vi "Serial_Port_Select.vi"(8 "error in":errorcluster, 11 "PortString":string) -> (0 "error out":errorcluster, 2 "SelectedPort":string, 3 "PortList":string[](array[string]))   [LabVIEW 2020]
uses:
  <vilib>/Instr/_visa.llb/VISA Find Search Mode.ctl
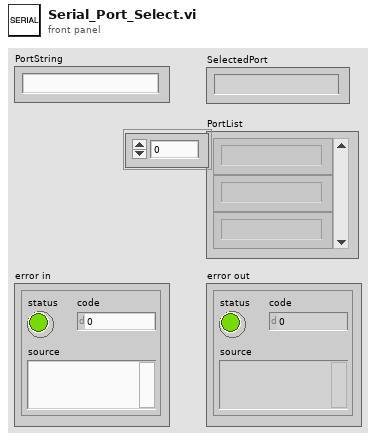
[diagram p1: front panel]
types:
  T1 = typedef "VISA Find Search Mode.ctl" = u32
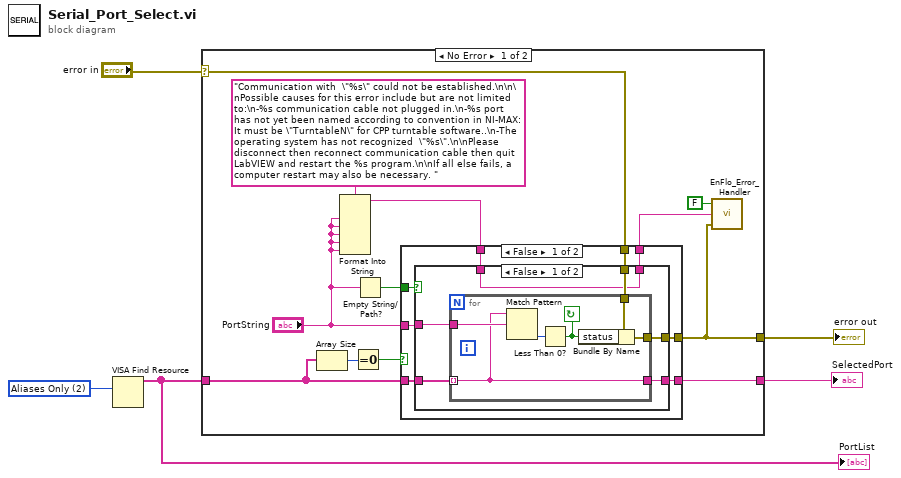
[diagram p0: block diagram]
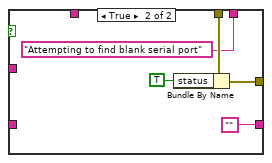
[diagram p2: hidden frame]
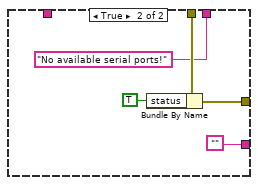
[diagram p3: hidden frame]
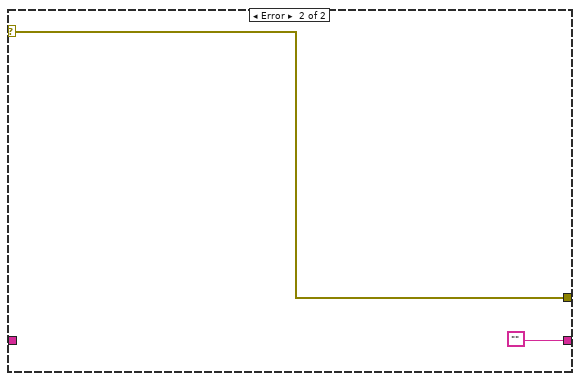
[diagram p4: hidden frame]
diagram:
  w2 = T1 2 items=["Canonical Names Only"=0, "Aliases Only"=2, "Include Matching Aliases"=3, "Include All Aliases"=4] ("Search Mode")
  n1 = VISA Find Resource(10:w2) -> (3:w1:string[])  [unwired: 1 in, 3 out]
  "PortList" <- w1
  n2 = case shown="No Error" "error in" {
    selector: "error in" -> [w14 w49]
    tunnel: [w17 ""] -> w5
    tunnel: [w16 w49] -> w4
    tunnel: w1 -> [w8 _]
    frame No Error {
      n3 = Array Size(array=w8) -> (size(s)=w7:i32)
      n4 = Format Into String(format string="Communication with  \"%s\" could not be established.\n\n\nPossible causes for this error include but are not limited to:\n-%s communication cable not plugged in.\n-%s port has not yet been named according to convention in NI-MAX: It must be \"TurntableN\" for CPP turntable software..\n-The operating system has not recognized  \"%s\".\n\nPlease disconnect then reconnect communication cable then quit LabVIEW and restart the %s program.\n\nIf all else fails, a computer restart may also be necessary. " ("string"), "PortString", "PortString", "PortString", "PortString", "PortString") -> (resulting string=w10:string)  [unwired: 2 in, 1 out]
      n5 = Equal To 0?(x=w7) -> (x = 0?=w6:bool)
      n6 = Empty String/Path?(string/path="PortString") -> (empty?=w11:bool)
      n7 = case shown="False" w6 {
        tunnel: [w25 ""] -> w17
        tunnel: [w24 w46] -> w16
        tunnel: w14 -> [w23 w47]
        tunnel: "PortString" -> [w22 _]
        tunnel: w11 -> [w21 _]
        tunnel: w10 -> [w20 _]
        tunnel: [w19 "No available serial ports!"] -> w9
        tunnel: w8 -> [w18 _]
        frame False {
          n8 = case shown="False" w21 {
            tunnel: [w27 ""] -> w25
            tunnel: [w31 w42] -> w24
            tunnel: w22 -> [w30 _]
            tunnel: w23 -> [w29 w41]
            tunnel: w18 -> [w28 _]
            tunnel: [w26 "Attempting to find blank serial port"] -> w19
            tunnel: w20 -> [w26 _]
            frame False {
              n9 = for {
                tunnel: w28 -> [w36] mode=indexing
                tunnel: w30 -> [w37]
                tunnel: [w36] -> w27
                tunnel: w29 -> [w35]
                tunnel: [w32] -> w31
                stop <- w33 continue-if-true
                n10 = Match Pattern(string=w36, regular expression=w37) -> (offset past match=w34:i32)  [unwired: 4 out]
                n11 = Less Than 0?(x=w34) -> (x < 0?=w33:bool)
                n12 = Bundle By Name(cluster=w35, "status"=w33) -> (w32:errorcluster)
              }
            }
            frame True {
              n13 = Bundle By Name(cluster=w41, "status"=TRUE) -> (w42:errorcluster)
            }
          }
        }
        frame True {
          n14 = Bundle By Name(cluster=w47, "status"=TRUE) -> (w46:errorcluster)
        }
      }
      n15 = call "EnFlo_Error_Handler.vi"("error in (no error)"=w16, "Error Type"=w9, "Dialog Box (F)"=FALSE) -> ()  [unwired: 1 in, 2 out]
    }
    frame Error {
    }
  }
  "SelectedPort" <- w5
  "error out" <- w4
